vi "Obtain.vi"(8 "error in (no error)":errorcluster, 11 "ID":i32) -> (0 "error out":errorcluster, 3 "Module":T1)   [LabVIEW 2022 SP3, in "Core.lvlib" / "Module.lvlib"]
uses:
  Module.lvlib
  Controls/Instance.ctl
  Controls/Module.ctl
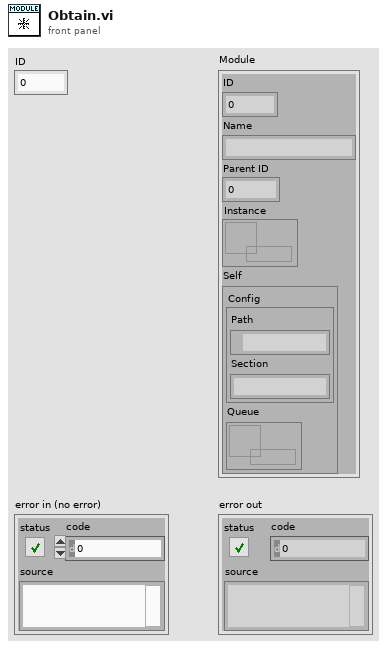
[diagram p1: front panel]
types:
  T1 = typedef "Core.lvlib/Module.lvlib/Module.ctl" = cluster{"ID":i32, "Name":string, "Parent ID":i32, "Instance":refnum<data-value>, "Self":T2}
  T2 = typedef "Core.lvlib/Module.lvlib/Instance.ctl" = cluster{"Config":cluster{"Path":path, "Section":string}, "Queue":refnum<queue>}
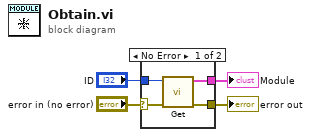
[diagram p0: block diagram]
diagram:
  n1 = case shown="No Error" "error in (no error)" {
    selector: "error in (no error)" -> [w8 w9]
    tunnel: [w7 w9] -> w3
    tunnel: "ID" -> [w6 _]
    tunnel: [w5 _] -> w1
    frame No Error {
      n2 = call "Get.vi"("error in (no error)"=w8, "ID"=w6) -> ("error out"=w7:errorcluster, "Module"=w5:T1)  [unwired: 8 in]
    }
    frame Error {
    }
  }
  "error out" <- w3
  "Module" <- w1
